vi "Definition Cluster.vi"(11 "Type in":refnum<class "Type.lvclass">) -> (2 "Definition":variant, 3 "Type out":refnum<class "Type.lvclass">)   [LabVIEW 2020, in "Conditu2.lvlib" / "Columns.lvlib" / "Type.lvclass"]
uses:
  Type.lvclass
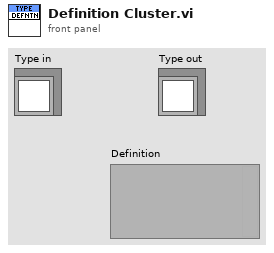
[diagram p1: front panel]
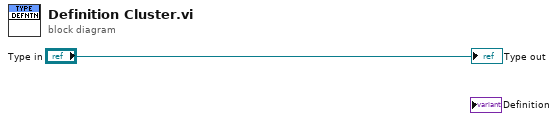
[diagram p0: block diagram]
diagram:
  "Type out" <- "Type in"
